vi "sv_Resize Plots in MSG.vi"(8 "error in (no error)":errorcluster, 9 "fractions of pixels":dbl[](array[numeric])=[0.5, 0.5], 10 "NewBnds":T2, 11 "array of control references in":refnum<vi>[](array[refnum])) -> (0 "error out":errorcluster, 2 "control dimensions":T1, 3 "array of control references out":refnum<vi>[](array[refnum]))   [LabVIEW 2017]
uses:
  <vilib>/Utility/miscctls.llb/LVRectTypeDef.ctl
  <vilib>/Utility/miscctls.llb/LVBoundsTypeDef.ctl
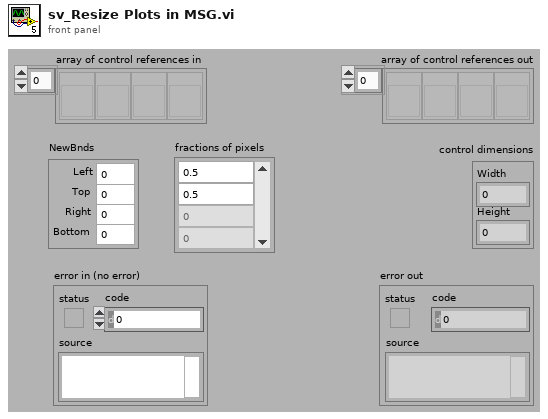
[diagram p1: front panel]
types:
  T1 = typedef "LVBoundsTypeDef.ctl" = cluster{"Width":u32, "Height":u32}
  T2 = typedef "LVRectTypeDef.ctl" = cluster{"Left":i16, "Top":i16, "Right":i16, "Bottom":i16}
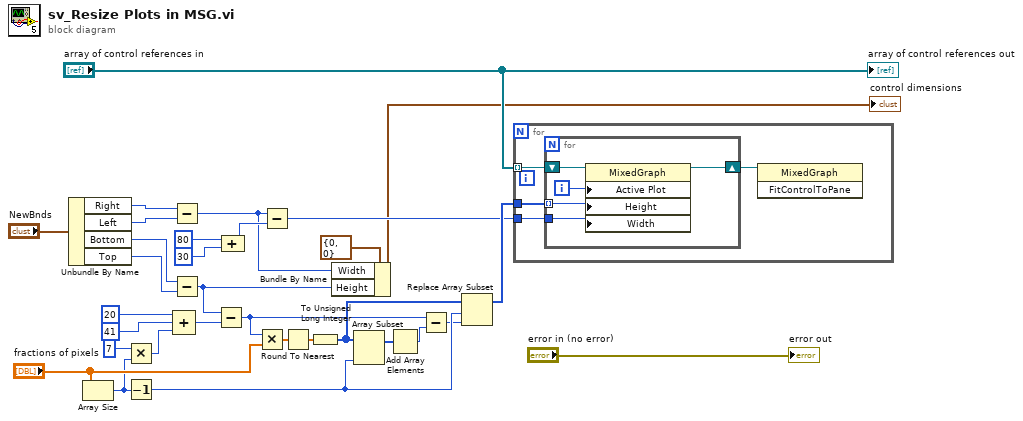
[diagram p0: block diagram]
diagram:
  n1 = Unbundle By Name("NewBnds") -> ("Right"=w14:i16, "Left"=w13:i16, "Bottom"=w25:i16, "Top"=w26:i16)
  n2 = Array Size(array="fractions of pixels") -> (size(s)=w6:i32)
  n3 = Multiply(x=u32 7 ("Active Plot Area"), y=w6) -> (x*y=w5:u32)
  n4 = Decrement(x=w6) -> (x-1=w21:i32)
  n5 = Subtract(x=w14, y=w13) -> (x-y=w2:i16)
  n6 = Subtract(x=w25, y=w26) -> (x-y=w1:i16)
  n7 = Compound Arithmetic op=ADD(u32 20 ("Active Plot Area"), u32 41 ("Active Plot Area"), w5) -> (w29:u32)
  n8 = Subtract(x=w1, y=w29) -> (x-y=w18:u32)
  n9 = Compound Arithmetic op=unknown(u32 80 ("Active Plot Area"), u32 30 ("Active Plot Area")) -> (w10:u32)
  n10 = Multiply(x=w18, y="fractions of pixels") -> (x*y=w24:dbl[])
  n11 = Subtract(x=w2, y=w10) -> (x-y=w9:u32)
  n12 = Round To Nearest(number=w24) -> (nearest integer value=w23:dbl[])
  n13 = To Unsigned Long Integer(number=w23) -> (unsigned 32bit integer=w22:u32[])
  n14 = Bundle By Name(cluster=T1 {"Width"=0, "Height"=0} ("Tab Control Pane Dimension"), "Width"=w2, "Height"=w1) -> (→"control dimensions":T1)
  n15 = Array Subset(array=w22, length=w21) -> (w19:u32[])  [unwired: 1 in]
  n16 = Add Array Elements(numeric array=w19) -> (sum=w17:u32)
  n17 = Subtract(x=w18, y=w17) -> (x-y=w16:u32)
  n18 = Replace Array Subset(array=w22, new element=w16, index=w21) -> (w15:u32[])
  n19 = for {
    tunnel: "array of control references in" -> [w35] mode=indexing
    tunnel: w15 -> [w34]
    tunnel: w9 -> [w33]
    n20 = for {
      shift-right: [w39] -> w32
      shift-left: w35 -> [w40]
      tunnel: w34 -> [w37] mode=indexing
      tunnel: w33 -> [w36]
      i -> [w38]
      n21 = property class="MixedGraph"(reference=w40, "Active Plot"=w38, "Height"=w37, "Width"=w36) -> (reference out=w39:refnum<vi>)  [unwired: 1 in, 1 out]
    }
    n22 = invoke class="MixedGraph" method="FitControlToPane"(reference=w32) -> ()  [unwired: 2 in, 3 out]
  }
  "array of control references out" <- "array of control references in"
  "error out" <- "error in (no error)"
